vi "HexStringToU8.vi"(0 "Input String":string, 7 "Starting Offset":i32) -> (4 "Number Out":u8)   [LabVIEW 2016]
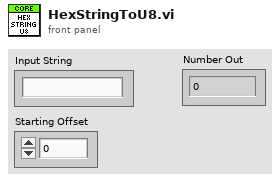
[diagram p1: front panel]
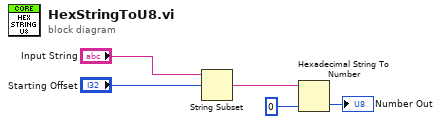
[diagram p0: block diagram]
diagram:
  n1 = String Subset(string="Input String", offset (0)="Starting Offset") -> (substring=w2:string)  [unwired: 1 in]
  n2 = Hexadecimal String To Number(string=w2, default (0uL)=u8 0) -> (number=→"Number Out":u8)  [unwired: 1 in, 1 out]
